vi "SIMPLE1.vi"() -> ()   [LabVIEW 2015]
panel:
  in  "file path comp X datta":path
  in  "file path joystick Y data":path
  in  "file path joystick X data":path
  in  "file path comp Y data":path
  out "XY JOYSTICK":cluster{"X":dbl[], "Y":dbl[]}[](graph)
  out "Y Array":u32[](array[numeric])
  out "XArray":u32[](array[numeric])
  out "XY Graph":cluster{"X":dbl[], "Y":dbl[]}[](graph)
  out "Y Array":u32[](array[numeric])
  out "X Array":u32[](array[numeric])
  in  "+X axis 2":bool
  out "code display 3":string
  in  "-X axis 2":bool
  in  "stop":bool
  in  "JOYSTICK":bool
  in  "SPEED":dbl(knob) scale=0.0..10.0
  in  "ACCELERATION":dbl(knob) scale=0.0..10.0
  in  "-Y axis":bool
  out "code display":string
  in  "+ Y axis":bool
  # "ENABLE"
  # "DISABLE"
  # "E X1 MN A1 V5 D-25000 G"
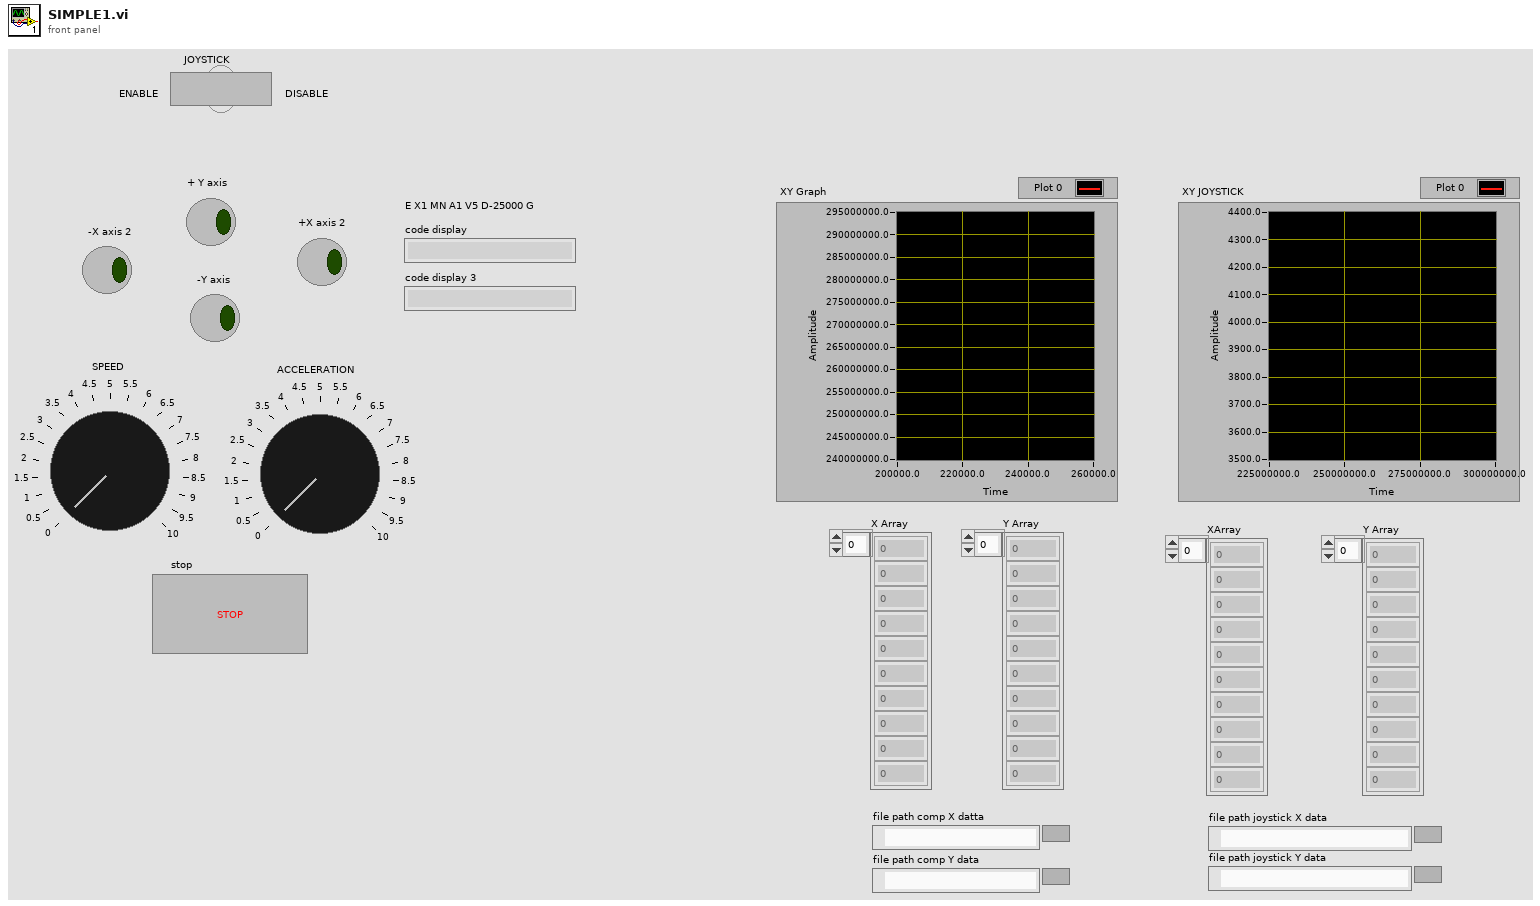
[diagram p1: front panel]
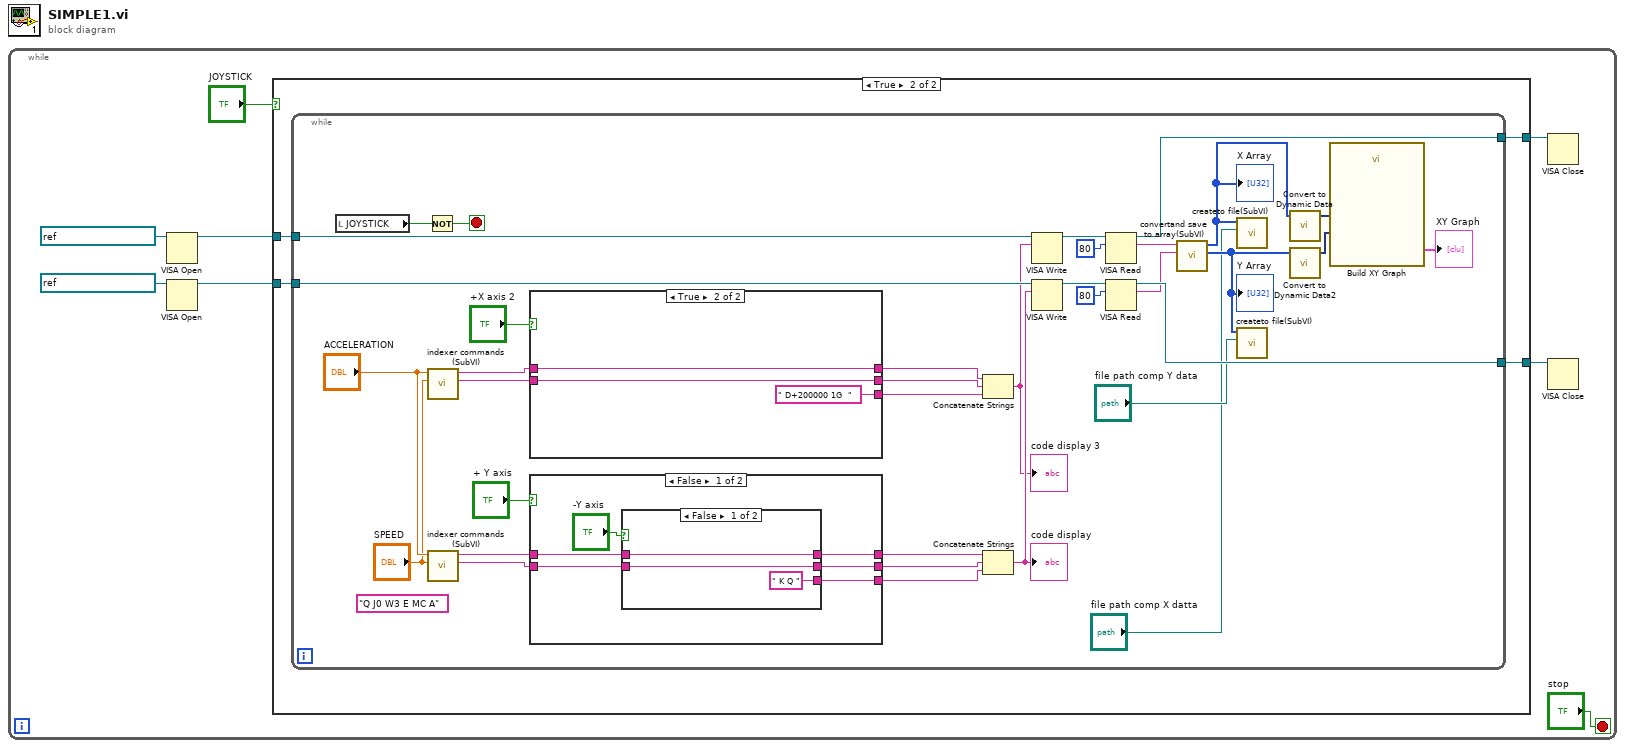
[diagram p0: block diagram]
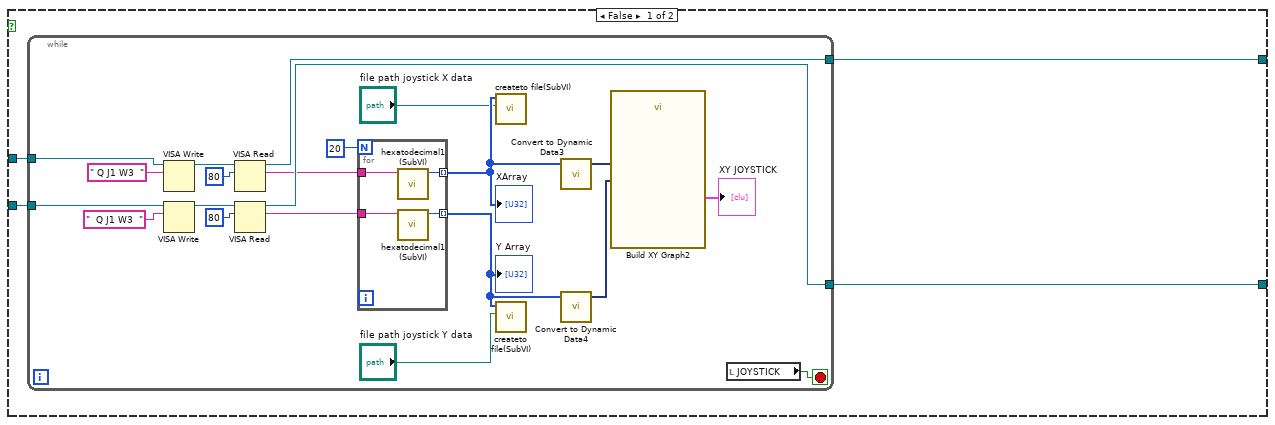
[diagram p2: hidden frame]
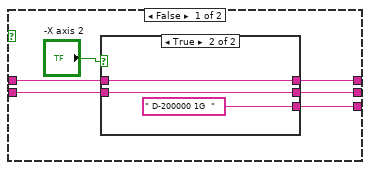
[diagram p3: hidden frame]
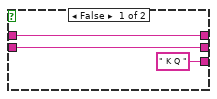
[diagram p4: hidden frame]
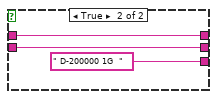
[diagram p5: hidden frame]
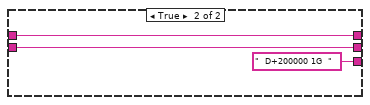
[diagram p6: hidden frame]
diagram:
  n1 = while {
    stop <- "stop" stop-if-true
    n2 = VISA Open(VISA resource name=refnum<visa-resource-name> "GPIB0::15::INSTR") -> (VISA resource name=w3:refnum<visa-resource-name>)  [unwired: 4 in, 1 out]
    n3 = VISA Open(VISA resource name=refnum<visa-resource-name> "GPIB0::16::INSTR") -> (VISA resource name=w7:refnum<visa-resource-name>)  [unwired: 4 in, 1 out]
    n4 = case shown="True" "JOYSTICK" {
      tunnel: w7 -> [w12 w41]
      tunnel: [w11 w38] -> w1
      tunnel: w3 -> [w9 w40]
      tunnel: [w10 w39] -> w2
      frame False {
        n5 = while {
          tunnel: w12 -> [w32]
          tunnel: [w25] -> w11
          tunnel: [w26] -> w10
          tunnel: w9 -> [w27]
          stop <- w31 stop-if-true
          n6 = VISA Write(VISA resource name=w27, write buffer=" Q J1 W3  ") -> (VISA resource name out=w28:refnum<visa-resource-name>)  [unwired: 1 in, 2 out]
          n7 = VISA Write(VISA resource name=w32, write buffer="  Q J1 W3  ") -> (VISA resource name out=w33:refnum<visa-resource-name>)  [unwired: 1 in, 2 out]
          n8 = VISA Read(VISA resource name=w28, byte count=u32 80) -> (VISA resource name out=w26:refnum<visa-resource-name>, read buffer=w21:string)  [unwired: 1 in, 2 out]
          n9 = VISA Read(VISA resource name=w33, byte count=u32 80) -> (VISA resource name out=w25:refnum<visa-resource-name>, read buffer=w20:string)  [unwired: 1 in, 2 out]
          n10 = for {
            N: 20 -> [_]
            tunnel: [w37] -> w16 mode=indexing
            tunnel: [w36] -> w15 mode=indexing
            tunnel: w21 -> [w35]
            tunnel: w20 -> [w34]
            n11 = call "hexatodecimal1 (SubVI).vi"("string in"=w35) -> ("Numeric"=w37:u32)  [unwired: 10 in]
            n12 = call "hexatodecimal1 (SubVI).vi"("string in"=w34) -> ("Numeric"=w36:u32)  [unwired: 10 in]
          }
          "XArray" <- w16
          "Y Array" <- w15
          n13 = call "createto file(SubVI).vi"("file path (use dialog) in"="file path joystick X data", "Array"=w16) -> ()  [unwired: 10 in]
          n14 = call "createto file(SubVI).vi"("file path (use dialog) in"="file path joystick Y data", "Array"=w15) -> ()  [unwired: 10 in]
          n15 = call "Convert to Dynamic Data3"("Array"=w16) -> ("Dynamic Data Type"=w18:dynamicdata)  [unwired: 3 in]
          n16 = call "Convert to Dynamic Data4"("Array"=w15) -> ("Dynamic Data Type"=w17:dynamicdata)  [unwired: 3 in]
          n17 = call "Build XY Graph2"("Y Input"=w17, "X Input"=w18) -> ("XY Graph"=→"XY JOYSTICK":cluster{"X":dbl[], "Y":dbl[]}[])  [unwired: 8 in, 1 out]
          n18 = local read "JOYSTICK"() -> (w31:bool)
        }
      }
      frame True {
        n19 = while {
          tunnel: w41 -> [w76]
          tunnel: [w73] -> w38
          tunnel: w40 -> [w72]
          tunnel: [w71] -> w39
          stop <- w74 stop-if-true
          (unwired) "Q J0 W3 E MC A" ("initial string")
          n20 = local read "JOYSTICK"() -> (w75:bool)
          n21 = Not(x=w75) -> (.not. x?=w74:bool)
          n22 = call "indexer commands (SubVI).vi"("SPEED"="SPEED", "ACCELERATION"="ACCELERATION") -> ("String"=w58:string, "String 2"=w59:string)  [unwired: 8 in]
          n23 = call "indexer commands (SubVI).vi"("SPEED"="SPEED", "ACCELERATION"="ACCELERATION") -> ("String"=w44:string, "String 2"=w45:string)  [unwired: 8 in]
          n24 = case shown="True" "+X axis 2" {
            tunnel: [w77 " D+200000 1G  " ("string")] -> w60
            tunnel: [w81 w89] -> w57
            tunnel: w59 -> [w80 w89]
            tunnel: w58 -> [w79 w90]
            tunnel: [w78 w90] -> w56
            frame False {
              n25 = case shown="True" "-X axis 2" {
                tunnel: [w85 w88] -> w81
                tunnel: w80 -> [w85 w88]
                tunnel: [w84 w87] -> w78
                tunnel: w79 -> [w84 w87]
                tunnel: [" K Q " ("string") " D-200000 1G  " ("string")] -> w77
                frame False {
                }
                frame True {
                }
              }
            }
            frame True {
            }
          }
          n26 = case shown="False" "+ Y axis" {
            tunnel: [w92 "  D+200000 1G  " ("string")] -> w65
            tunnel: [w96 w104] -> w64
            tunnel: w45 -> [w95 w104]
            tunnel: w44 -> [w94 w105]
            tunnel: [w93 w105] -> w63
            frame False {
              n27 = case shown="False" "-Y axis" {
                tunnel: [w100 w103] -> w96
                tunnel: w95 -> [w100 w103]
                tunnel: [w99 w102] -> w93
                tunnel: w94 -> [w99 w102]
                tunnel: [" K Q " ("string") " D-200000 1G  " ("string")] -> w92
                frame False {
                }
                frame True {
                }
              }
            }
            frame True {
            }
          }
          n28 = Concatenate Strings(w57, w56, w60) -> (w61:string)
          "code display 3" <- w61
          n29 = Concatenate Strings(w64, w63, w65) -> (w66:string)
          "code display" <- w66
          n30 = VISA Write(VISA resource name=w72, write buffer=w61) -> (VISA resource name out=w69:refnum<visa-resource-name>)  [unwired: 1 in, 2 out]
          n31 = VISA Write(VISA resource name=w76, write buffer=w66) -> (VISA resource name out=w70:refnum<visa-resource-name>)  [unwired: 1 in, 2 out]
          n32 = VISA Read(VISA resource name=w69, byte count=u32 80) -> (VISA resource name out=w71:refnum<visa-resource-name>, read buffer=w68:string)  [unwired: 1 in, 2 out]
          n33 = VISA Read(VISA resource name=w70, byte count=u32 80) -> (VISA resource name out=w73:refnum<visa-resource-name>, read buffer=w67:string)  [unwired: 1 in, 2 out]
          n34 = call "convertand save to array(SubVI).vi"("read buffer"=w67, "read buffer 2"=w68) -> ("Array 2"=w48:u32[], "Array"=w47:u32[])  [unwired: 8 in]
          "X Array" <- w47
          "Y Array" <- w48
          n35 = call "createto file(SubVI).vi"("file path (use dialog) in"="file path comp X datta", "Array"=w47) -> ()  [unwired: 10 in]
          n36 = call "createto file(SubVI).vi"("file path (use dialog) in"="file path comp Y data", "Array"=w48) -> ()  [unwired: 10 in]
          n37 = call "Convert to Dynamic Data"("Array"=w47) -> ("Dynamic Data Type"=w51:dynamicdata)  [unwired: 3 in]
          n38 = call "Convert to Dynamic Data2"("Array"=w48) -> ("Dynamic Data Type"=w50:dynamicdata)  [unwired: 3 in]
          n39 = call "Build XY Graph"("Y Input"=w50, "X Input"=w51) -> ("XY Graph"=→"XY Graph":cluster{"X":dbl[], "Y":dbl[]}[])  [unwired: 8 in, 1 out]
        }
      }
    }
    n40 = VISA Close(VISA resource name=w2) -> ()  [unwired: 1 in, 1 out]
    n41 = VISA Close(VISA resource name=w1) -> ()  [unwired: 1 in, 1 out]
  }
